vi "Write Init VI Properties.vi"(8 "Error In":errorcluster, 10 "Initialization VI Properties":T1, 11 "Custom Device .NET Ref In":refnum<k24>) -> (0 "Error Out":errorcluster, 3 "Custom Device .NET Ref Out":refnum<k24>)   [LabVIEW 2015, in "VeriStand XML Parser.lvlib"]
doc: "Writes the properties of the custom device initialization VI"
uses:
  VeriStand XML Parser.lvlib
  NationalInstruments.VeriStand.XMLReader
  XML Controls/Initialization VI Properties.ctl
  XML Controls/Execution Types.ctl
  XML Controls/Path Cluster.ctl
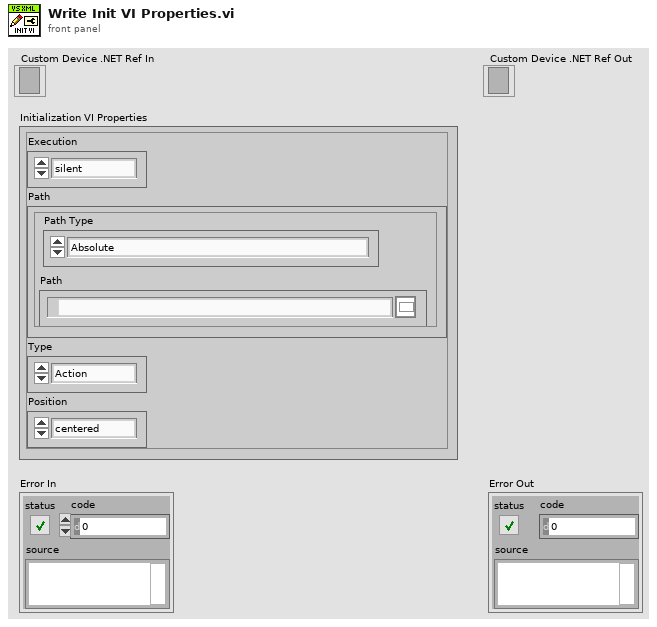
[diagram p1: front panel]
types:
  T1 = typedef "VeriStand XML Parser.lvlib/Initialization VI Properties.ctl" = cluster{"Execution":T2, "Path":T3, "Type":enum16{"Action", "VI"}, "Position":enum16{"centered", "mouse pointer"}}
  T2 = typedef "VeriStand XML Parser.lvlib/Execution Types.ctl" = enum16{"silent", "modal", "floating", "default"}
  T3 = typedef "VeriStand XML Parser.lvlib/Path Cluster.ctl" = cluster{"Path":path, "Path Type":enum16{"Absolute", "To Base", "To Common Doc Dir", "To Application Data Dir"}}
  T4 = enum16{"Absolute", "To Base", "To Common Doc Dir", "To Application Data Dir"}
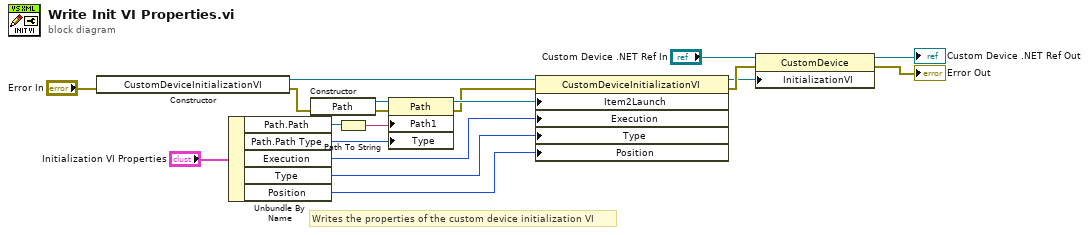
[diagram p0: block diagram]
diagram:
  # "Writes the properties of the custom device initialization VI"
  n1 = constructor class="CustomDeviceInitializationVI"(error in="Error In") -> (reference out=w3:refnum<k24>, error out=w6:errorcluster)  [unwired: 2 in, 1 out]
  n2 = Unbundle By Name("Initialization VI Properties") -> ("Path.Path"=w9:path, "Path.Path Type"=w11:T4, "Execution"=w12:T2, "Type"=w13:enum16{"Action", "VI"}, "Position"=w14:enum16{"centered", "mouse pointer"})
  n3 = constructor class="Path"(error in=w6) -> (reference out=w5:refnum<k24>, error out=w4:errorcluster)  [unwired: 2 in, 1 out]
  n4 = Path To String(path=w9) -> (string=w10:string)
  n5 = property class="Path"(reference=w5, error in=w4, "Path1"=w10, "Type"=w11) -> (reference out=w8:refnum<k24>, error out=w7:errorcluster)
  n6 = property class="CustomDeviceInitializationVI"(reference=w3, error in=w7, "Item2Launch"=w8, "Execution"=w12, "Type"=w13, "Position"=w14) -> (reference out=w16:refnum<k24>, error out=w17:errorcluster)
  n7 = property class="CustomDevice"(reference="Custom Device .NET Ref In", error in=w17, "InitializationVI"=w16) -> (reference out=→"Custom Device .NET Ref Out":refnum<k24>, error out=→"Error Out":errorcluster)
